vi "Add Branch to Tree.vi"(6 "Truncate Branch?":bool=TRUE, 8 "error in":errorcluster, 9 "Branch in":refnum<class "Tree.lvclass">, 11 "Root in":refnum<class "Tree.lvclass">) -> (0 "error out":errorcluster, 1 "Branch out":refnum<class "Tree.lvclass">, 3 "Root out":refnum<class "Tree.lvclass">)   [LabVIEW 2019, in "Tree.lvclass"]
uses:
  Tree.lvclass
  Tree.lvclass/Tree.ctl
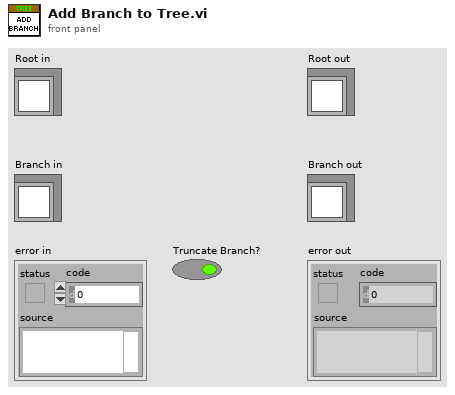
[diagram p1: front panel]
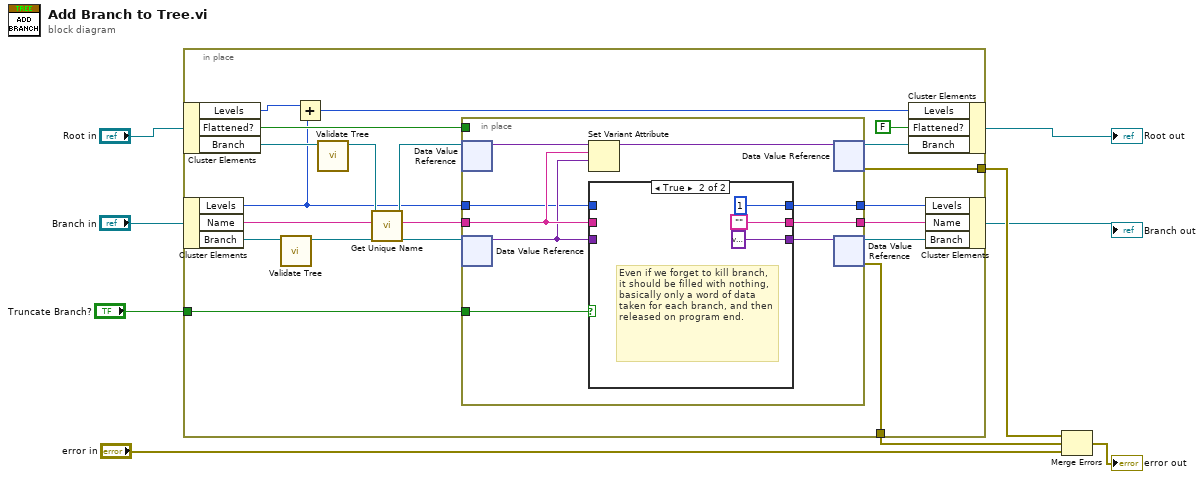
[diagram p0: block diagram]
diagram:
  n1 = in-place {
    in-place-border: [w27] -> w6
    in-place-border: [w16] -> w3
    in-place-border: "Truncate Branch?" -> [w12]
    n2 = in-place-cluster #1("Root in") -> ("Levels"=w14:u32, "Flattened?"=w15:bool, "Branch"=w19:refnum<data-value>)
    n3 = in-place-cluster #2("Branch in") -> ("Levels"=w10:u32, "Name"=w23:string, "Branch"=w18:refnum<data-value>)
    n4 = call "Validate Tree.vi"("Branch Reference In"=w18) -> ("Branch Reference Out"=w17:refnum<data-value>)  [unwired: 9 in, 1 out]
    n5 = Add(x=w14, y=w10) -> (x+y=w13:u32)
    n6 = call "Validate Tree.vi"("Branch Reference In"=w19) -> ("Branch Reference Out"=w20:refnum<data-value>)  [unwired: 9 in, 1 out]
    n7 = call "Get Unique Name.vi"("Name"=w23, "Branch"=w20) -> ("Unique Name"=w22:string, "Branch"=w24:refnum<data-value>)  [unwired: 7 in, 1 out]
    n8 = in-place {
      in-place-border: w22 -> [w32]
      in-place-border: [w34] -> w25
      in-place-border: w15 -> [_]
      in-place-border: w12 -> [w35]
      in-place-border: [w30] -> w11
      in-place-border: w10 -> [w29]
      n9 = in-place-dvr #3(w24) -> (w37:variant)  [unwired: 1 out]
      n10 = in-place-dvr #4(w17) -> (w31:variant)  [unwired: 1 out]
      n11 = Set Variant Attribute(Variant=w37, name=w32, value=w31) -> (Variant out=w36:variant)  [unwired: 1 in, 2 out]
      n12 = case shown="True" w35 {
        tunnel: [w40 ""] -> w34
        tunnel: [w39 variant ("data value")] -> w33
        tunnel: w32 -> [w40 _]
        tunnel: w31 -> [w39 _]
        tunnel: [w38 u32 1 ("Levels")] -> w30
        tunnel: w29 -> [w38 _]
        frame False {
        }
        frame True {
          # "Even if we forget to kill branch, it should be filled with nothing, basically only a word of data taken for each branch, and then released on program end."
        }
      }
      n13 = in-place-dvr #3(w36) -> (w28:refnum<data-value>, w27:errorcluster)
      n14 = in-place-dvr #4(w33) -> (w26:refnum<data-value>, w16:errorcluster)
    }
    n15 = in-place-cluster #1("Levels"=w13, "Flattened?"=FALSE ("Flattened Up to Date?"), "Branch"=w28) -> (→"Root out":refnum<class "Tree.lvclass">)
    n16 = in-place-cluster #2("Levels"=w11, "Name"=w25, "Branch"=w26) -> (→"Branch out":refnum<class "Tree.lvclass">)
  }
  n17 = Merge Errors(w6, w3, "error in") -> (→"error out":errorcluster)
